vi "TCPClientCycle.vi"   [LabVIEW 2019]
uses:
  02 Mode/TCPClientMode/TCPClientClass.lvclass
types:
  T1 = map{string, refnum<class "TCPClientClass.lvclass">}
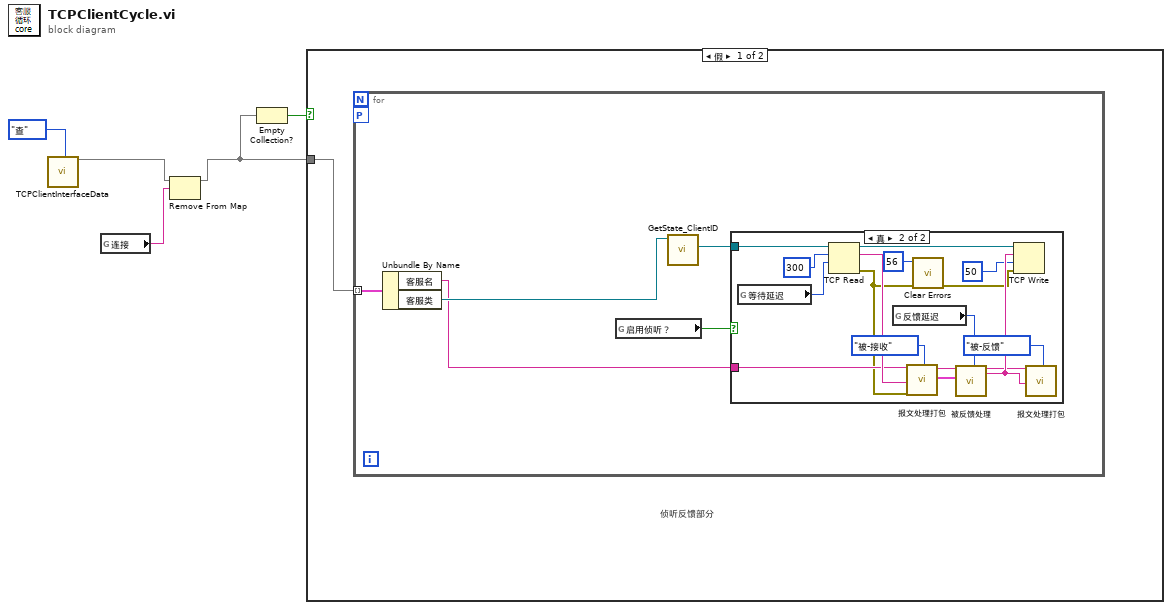
[diagram p0: block diagram]
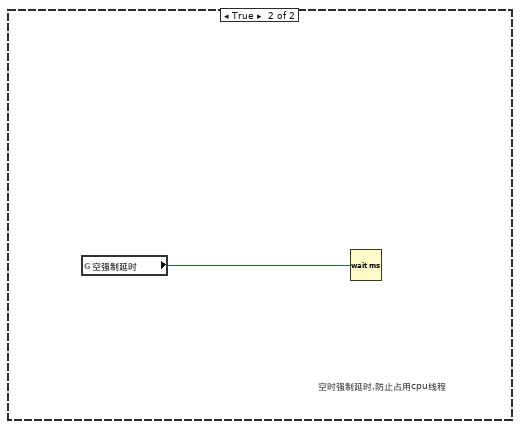
[diagram p3: hidden frame]
diagram:
  n1 = call "TCPClientInterfaceData.vi"("客服接口枚举"=enum16{"ini", "增", "删", "查", "改"}."查") -> ("客服表"=w3:T1)  [unwired: 17 in, 1 out]
  n2 = global read "全局-配置识别.vi" "连接"() -> (w2:string)
  n3 = Remove From Map(10:w2, 11:w3) -> (3:w1:T1)  [unwired: 2 out]
  n4 = Empty Collection?(1:w1) -> (0:w5:bool)
  n5 = case shown="假" w5 {
    tunnel: w1 -> [w6 _]
    frame False {
      # "侦听反馈部分"
      n6 = for {
        tunnel: w6 -> [w11] mode=indexing
        workers-P: _ -> [_]
        n7 = Unbundle By Name(w11) -> ("客服名"=w9:string, "客服类"=w10:refnum<class "TCPClientClass.lvclass">)
        n8 = global read "全局-被反馈配置.vi" "启用侦听？"() -> (w7:bool)
        n9 = call-dynamic "GetState_ClientID.vi"("TCPClientClass输入"=w10) -> ("连接ID"=w8:refnum<k5>)  [unwired: 8 in, 2 out]
        n10 = case shown="真" w7 {
          tunnel: w8 -> [_ w28]
          tunnel: w9 -> [_ w22]
          frame False {
          }
          frame True {
            n11 = global read "全局-配置识别.vi" "等待延迟"() -> (w27:u32)
            n12 = TCP Read(connection ID=w28, bytes to read=300 ("读取的字节"), 9:w27) -> (connection ID out=w12:refnum<k5>, data out=w24:string, error out=w15:errorcluster)  [unwired: 2 in]
            n13 = global read "全局-配置识别.vi" "反馈延迟"() -> (w16:u32)
            n14 = call "报文处理打包.vi"("识别名称"=w22, "报文"=w24, "Error In"=w15, "类型"=enum16{"被-接收", "被-反馈", "主-发", "主-收"}."被-接收") -> ("识别名称输出"=w20:string, "被收校验信息"=w19:cluster{"可用？":bool, "功能码":u8, "无crc报文":u8[]})  [unwired: 14 in]
            n15 = call <vilib>:"Clear Errors.vi"("error in (no error)"=w15, "specific error code to clear (0: all)"=56) -> ("error out"=w13:errorcluster)  [unwired: 4 in, 1 out]
            n16 = call "被反馈处理.vi"("识别名称"=w20, "校验信息"=w19, "等待时间（毫秒）"=w16) -> ("识别名称输出"=w18:string, "反馈"=w25:string)  [unwired: 15 in]
            n17 = TCP Write(connection ID=w12, data in=w25, error in (no error)=w13, 9:50 ("超时毫秒(25000)")) -> ()  [unwired: 3 out]
            n18 = call "报文处理打包.vi"("识别名称"=w18, "报文"=w25, "类型"=enum16{"被-接收", "被-反馈", "主-发", "主-收"}."被-反馈") -> ()  [unwired: 15 in, 2 out]
          }
        }
      }
    }
    frame True {
      # "空时强制延时,防止占用cpu线程"
      n19 = global read "全局-配置识别.vi" "空强制延时"() -> (w29:u32)
      n20 = Wait (ms)(milliseconds to wait=w29) -> ()  [unwired: 1 out]
    }
  }
